vi "Test DBL Omnibus Event.vi"() -> ()   [LabVIEW 2021]
uses:
  Source/Omni-Bus/Omni_Bus.lvclass
  Source/Event Bus/Event_Bus.lvclass
  C:/TSA/Omni-Bus/Source/Omni-Bus/Bus Access/Bus_Access.lvclass
  Source/Local Bus/Local Bus.lvclass
  Source/Omni-Bus/Support/Broad Types.ctl
  Source/Event Bus/Support/Event Source/Polled_EventSource/Polled_EventSource.lvclass
  C:/TSA/Omni-Bus/Source/Event Bus/Support/Event Source/Event_Source.lvclass
  Source/Local Bus/Support/Tag List Type.ctl
  <vilib>/Utility/Data Type/Type Definitions/Data Type.ctl
  <vilib>/TSA/Abstract Data Classes/Abs_Types/Type/Abs_Type.lvclass/Abs_Type.ctl
  Source/Omni-Bus/Omni_Bus.lvclass/Omni_Bus.ctl
  Source/Omni-Bus/Support/Write/Write DBL.vi
  Source/Omni-Bus/Support/Read/Read DBL.vi
  Source/Omni-Bus/Support/FindVar.vi
  <vilib>/Utility/error.llb/Clear Errors.vi
  <vilib>/TSA/Abstract Data Classes/Abs_Types/Type/Properties/Write Tag.vi
  Source/Omni-Bus/Properties/Read Var Map.vi
  <vilib>/TSA/Abstract Data Classes/Abs_Types/Type/Properties/Read Tag.vi
  <vilib>/TSA/Abstract Data Classes/Abs_Types/Double Float/Abs_Double Float.lvclass
  C:/Program Files (x86)/National Instruments/LabVIEW 2021/vi.lib/TSA/Abstract Data Classes/Abs_Types/Type/Abs_Type.lvclass
  <vilib>/TSA/Abstract Data Classes/Abs_Types/Value/Abs_Value.lvclass
  Source/Omni-Bus/Support/Check For Read Only Error.vi
  Source/Omni-Bus/Support/Incorrect Tag String Error.vi
  <vilib>/TSA/Abstract Data Classes/Abs_Types/Type/Abs_Type.lvclass
  <vilib>/Utility/Data Type/NI_Data Type.lvlib
  <vilib>/ptbypt/NI_PtbyPt.lvlib
panel:
  out "Waveform Chart":dbl(graph)
  in  "Combo Box 3":string(combo)
  in  "Combo Box 2":string(combo)
  in  "Combo Box":string(combo)
  in  "stop 6":bool
  out "Numeric 6":i32
  in  "Numeric 5":dbl
  out "Numeric 3":dbl
  out "Numeric 2":i32
  out "Numeric":i32
  in  "stop 2":bool
  in  "stop":bool
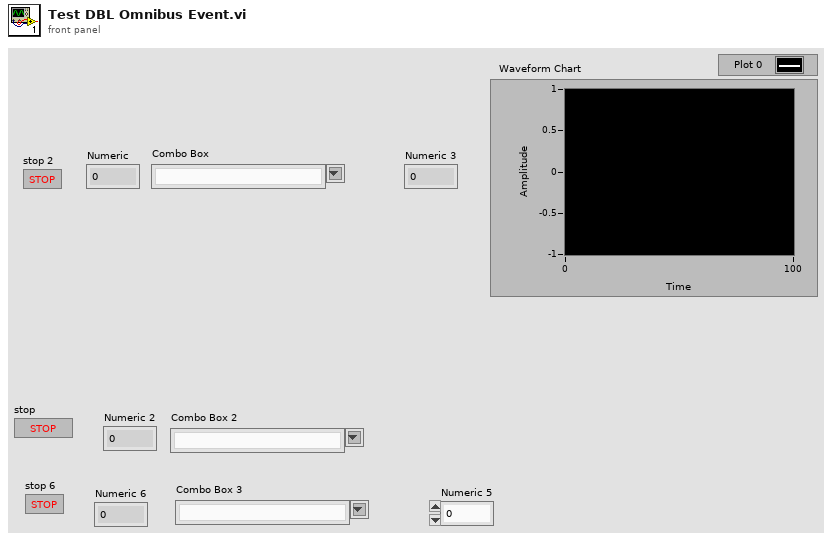
[diagram p1: front panel]
types:
  T1 = typedef "Omni_Bus.lvclass/Broad Types.ctl" = enum16{"All Tags", "NI Specific Type", "Boolean", "String", "Numeric", "Float", "Integer", "Collection", "All Value Types", "Non Value Types"}
  T2 = typedef "Local Bus.lvclass/Tag List Type.ctl" = cluster{"Tag":string, "Type":T3}
  T3 = typedef "NI_Data Type.lvlib/Data Type.ctl" = enum8{"Invalid Type", "Void", "I8", "I16", "I32", "I64", "U8", "U16", "U32", "U64", "Single Float", "Double Float", "Extended Float", "Single Complex", "Double Complex", "Extended Complex", "Enum U8", "Enum U16", "Enum U32", "Enum U64", "Single Float With Unit", "Double Float With Unit", "Extended Float With Unit", "Single Complex with Unit", "Double Complex with Unit", "Extended Complex with Unit", "Boolean", "String", "Path", "Picture", "Tag", "Array", "Cluster", "Variant", "LV Variant", "Waveform", "Timestamp", "Digital Waveform", "Digital Data", "ExpressData", "Refnum", "External Data", "VI", "Poly VI", "LabVIEW Class Instance", "Fixed Point", "Set Collection", "Map Collection"}
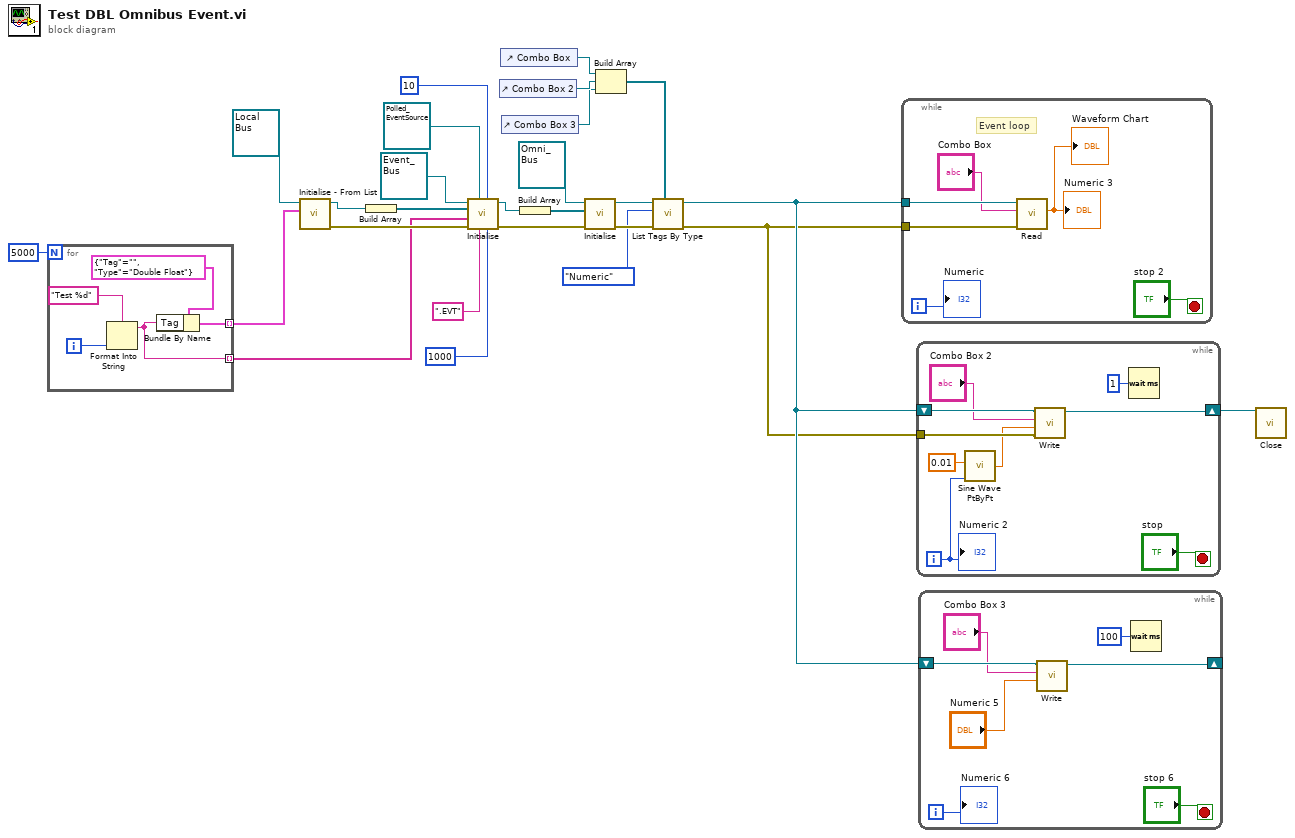
[diagram p0: block diagram]
diagram:
  n1 = for {
    N: 5000 -> [_]
    tunnel: [w28] -> w15 mode=indexing
    tunnel: [w27] -> w12 mode=indexing
    i -> [w29]
    n2 = Format Into String(format string="Test %d", w29) -> (resulting string=w27:string)  [unwired: 2 in, 1 out]
    n3 = Bundle By Name(cluster=T2 {"Tag"="", "Type"=enum."Double Float"} ("Cluster"), "Tag"=w27) -> (w28:T2)
  }
  n4 = call "Initialise - From List.vi"("Tag List"=w15, "Local Bus in"=refnum<class "Local Bus.lvclass"> refnum) -> ("error out"=w20:errorcluster, "Local Bus out"=w19:refnum<class "Local Bus.lvclass">)  [unwired: 8 in]
  n5 = Build Array(w19) -> (w21:refnum<class "Local Bus.lvclass">[])
  n6 = call "Initialise.vi"("Default Timeout (ms)"=1000, "Poll Interval (ms)"=10, "Tag Root"=".EVT", "Event_Source.lvclass"=refnum<class "Polled_EventSource.lvclass"> refnum ("Polled_EventSource.lvclass"), "error in (no error)"=w20, "Tags to Create Events For"=w12, "Buses"=w21, "Event_Bus in"=refnum<class "Event_Bus.lvclass"> refnum) -> ("error out"=w24:errorcluster, "Event_Bus out"=w23:refnum<class "Event_Bus.lvclass">)  [unwired: 2 in]
  n7 = control-ref of="Combo Box 2"() -> (w6:refnum<vi>)
  n8 = control-ref of="Combo Box"() -> (w7:refnum<vi>)
  n9 = control-ref of="Combo Box 3"() -> (w5:refnum<vi>)
  n10 = Build Array(w23) -> (w25:refnum<class "Event_Bus.lvclass">[])
  n11 = call-dynamic "Initialise.vi"("error in (no error)"=w24, "Bus Access"=w25, "Var Bus in"=refnum<class "Omni_Bus.lvclass"> refnum) -> ("error out"=w9:errorcluster, "Var Bus out"=w11:refnum<class "Omni_Bus.lvclass">)  [unwired: 7 in]
  n12 = Build Array(w7, w6, w5) -> (w4:refnum<vi>[])
  n13 = call "List Tags By Type.vi"("Combo Boxes"=w4, "error in (no error)"=w9, "Broad Types"=Broad_Types."Numeric", "Var Bus in"=w11) -> ("error out"=w8:errorcluster, "Var Bus out"=w10:refnum<class "Omni_Bus.lvclass">)  [unwired: 4 in, 2 out]
  n14 = while {
    tunnel: w10 -> [w37]
    tunnel: w8 -> [w36]
    i -> [w34]
    stop <- "stop 2" stop-if-true
    # "Event loop"
    n15 = call-poly "Read.vi"("error in (no error)"=w36, "Tag"="Combo Box", "Var Bus in"=w37) -> ("Numeric"=→"Numeric 3" →"Waveform Chart":dbl)  [unwired: 6 in, 2 out]
    "Numeric" <- w34
  }
  n16 = while {
    tunnel: w8 -> [w44]
    shift-right: [w43] -> w17
    shift-left: w10 -> [w45]
    i -> [w39]
    stop <- "stop" stop-if-true
    n17 = call <vilib>:"Sine Wave PtByPt.vi"("time"=w39, "frequency"=0.01) -> ("sine wave"=w40:dbl)  [unwired: 2 in]
    n18 = call-poly "Write.vi"("error in (no error)"=w44, "Numeric"=w40, "Tag"="Combo Box 2", "Omni_Bus in"=w45) -> ("Omni_Bus out"=w43:refnum<class "Omni_Bus.lvclass">)  [unwired: 6 in, 1 out]
    n19 = Wait (ms)(milliseconds to wait=u32 1) -> ()  [unwired: 1 out]
    "Numeric 2" <- w39
  }
  n20 = while {
    shift-right: [w49] -> _
    shift-left: w10 -> [w52]
    i -> [w51]
    stop <- "stop 6" stop-if-true
    n21 = call-poly "Write.vi"("Numeric"="Numeric 5", "Tag"="Combo Box 3", "Omni_Bus in"=w52) -> ("Omni_Bus out"=w49:refnum<class "Omni_Bus.lvclass">)  [unwired: 7 in, 1 out]
    n22 = Wait (ms)(milliseconds to wait=u32 100) -> ()  [unwired: 1 out]
    "Numeric 6" <- w51
  }
  n23 = call-dynamic "Close.vi"("Data in"=w17) -> ()  [unwired: 9 in, 2 out]
